vi "initialize_all_channels.vi"(8 "error in":errorcluster, 9 "id_in":i32, 11 "connection ID":refnum<k5>) -> (0 "error out":errorcluster, 1 "id_out":i32, 3 "connection ID out":refnum<k5>)   [LabVIEW 2009]
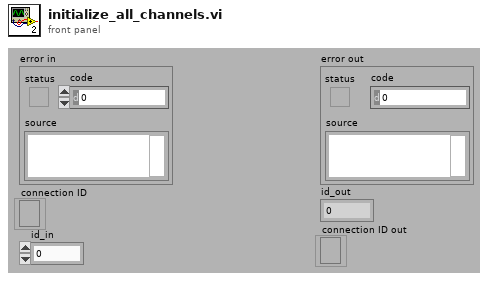
[diagram p1: front panel]
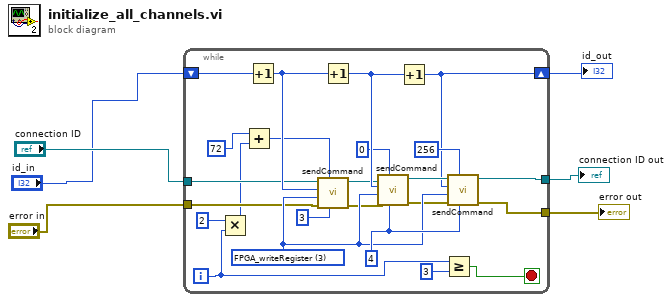
[diagram p0: block diagram]
diagram:
  n1 = while {
    tunnel: [w19] -> w6
    tunnel: [w18] -> w5
    tunnel: "connection ID" -> [w17]
    tunnel: "error in" -> [w16]
    shift-right: [w7] -> w1
    shift-left: "id_in" -> [w15]
    i -> [w12]
    stop <- w14 stop-if-true
    w26 = 4 ("Address")
    w24 = u16 3 items=["sendCommand"=9, "FPGA_writeRegister"=3, "FPGA_readRegister"=2, "uC_writeRegister"=1, "uC_readRegister"=0] ("Action")
    n2 = Multiply(x=2, y=w12) -> (x*y=w10:i32)
    n3 = Add(x=72 ("Data"), y=w10) -> (x+y=w8:i32)
    n4 = Increment(x=w15) -> (x+1=w29:i32)
    n5 = call "sendCommand.vi"("Address"=3, "Data"=w8, "error in"=w16, "Action"=w24, "id_in"=w29, "connection ID"=w17) -> ("error out"=w22:errorcluster, "connection ID out"=w20:refnum<k5>)  [unwired: 1 in, 3 out]
    n6 = Increment(x=w29) -> (x+1=w30:i32)
    n7 = call "sendCommand.vi"("Address"=w26, "Data"=0, "error in"=w22, "Action"=w24, "id_in"=w30, "connection ID"=w20) -> ("error out"=w23:errorcluster, "connection ID out"=w21:refnum<k5>)  [unwired: 1 in, 3 out]
    n8 = Increment(x=w30) -> (x+1=w7:i32)
    n9 = Greater Or Equal?(x=w12, y=3) -> (x >= y?=w14:bool)
    n10 = call "sendCommand.vi"("Address"=w26, "Data"=256, "error in"=w23, "Action"=w24, "id_in"=w7, "connection ID"=w21) -> ("error out"=w19:errorcluster, "connection ID out"=w18:refnum<k5>)  [unwired: 1 in, 3 out]
  }
  "error out" <- w6
  "id_out" <- w1
  "connection ID out" <- w5
